vi "Initialize RF boards - interlace 3 v2.vi"(2 "error in":errorcluster, 3 "FPGA VI Reference In":T1) -> (0 "error out":errorcluster, 1 "FPGA VI Reference Out":T1)   [LabVIEW 2012]
uses:
  <vilib>/rvi/interface/nirviReadWriteControl/nirviReadWriteControl.xnode
  openfpgaref.8.6.ctl
  NiFpgaLv.dll
  <vilib>/Utility/error.llb/Error Cluster From Error Code.vi
  <vilib>/rvi/errors/niLvFpgaAdjustHostInterfaceError.vi
  FPGA Bitfiles/UHR-FleezersInst_FPGATarget_UHR-Fleezers_main_12.5_v1.lvbitx
  <vilib>/rvi/errors/niLvFpgaMergeErrorWithErrorCode.vi
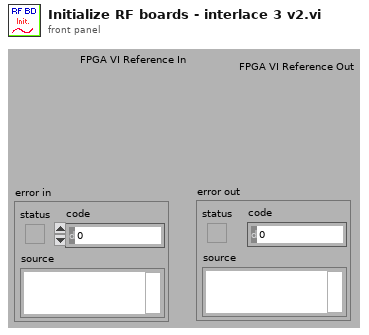
[diagram p1: front panel]
types:
  T1 = typedef "openfpgaref.8.6.ctl" = refnum<k20>
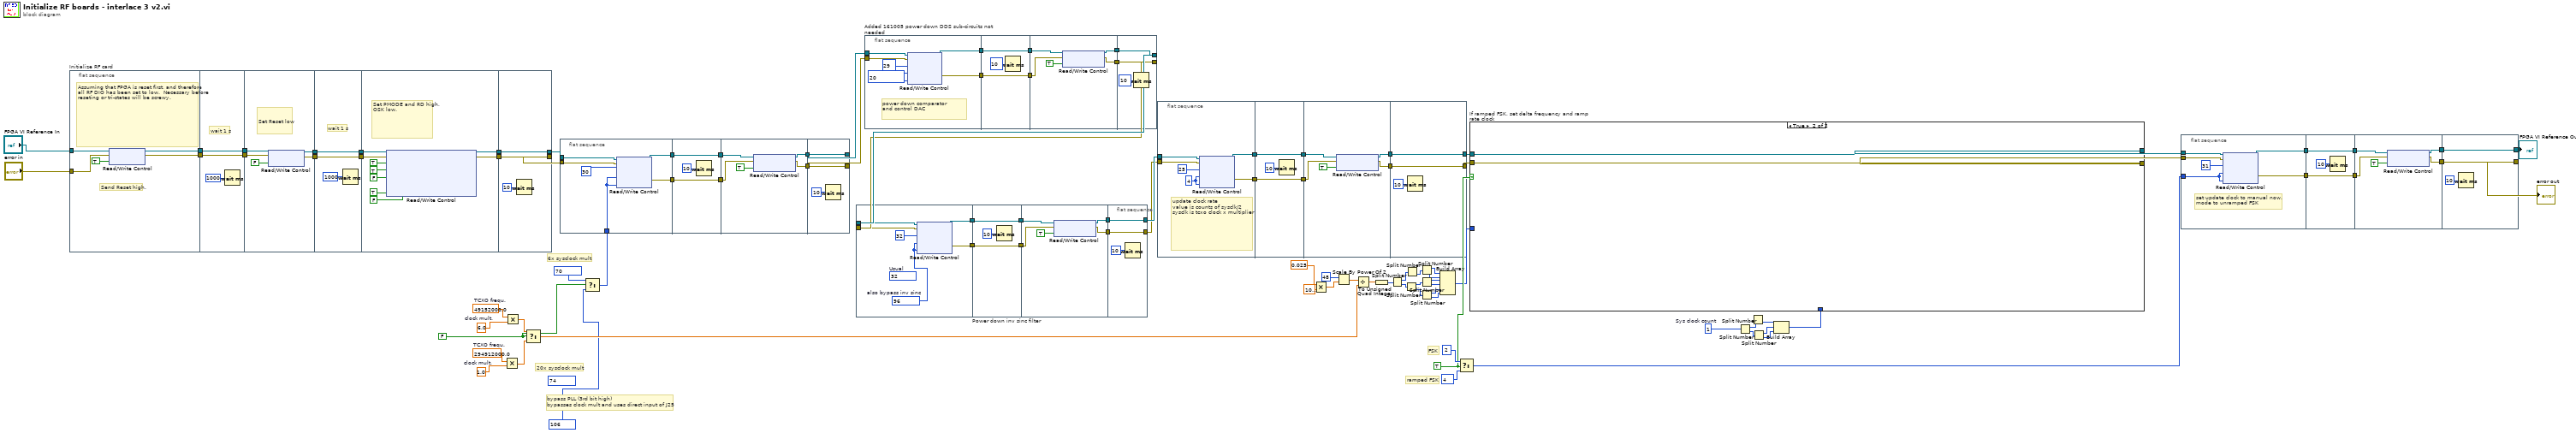
[diagram p0: block diagram]
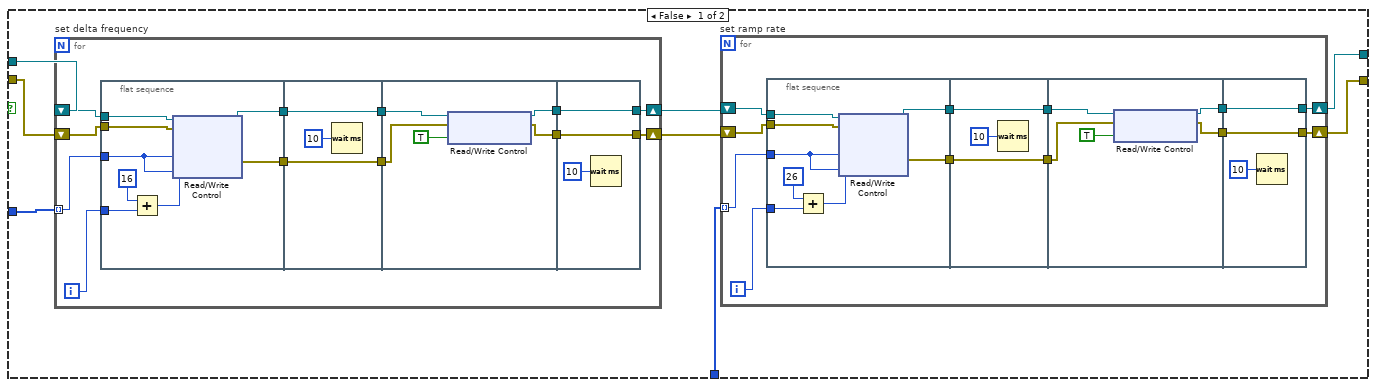
[diagram p2: hidden frame]
diagram:
  (unwired) u8 74 ("Data")
  w14 = FALSE ("s")
  w18 = 1.0  # clock mult.
  w17 = 294912000.0  # TCXO frequ.
  w21 = 6.0  # clock mult.
  w20 = 49152000.0  # TCXO frequ.
  w30 = u32 1  # Sys clock count
  w51 = TRUE
  # "bypass PLL (3rd bit high)\nbypasses clock mult and uses direct input of J25"
  # "20x sysclock mult"
  # "6x sysclock mult"
  # "ramped FSK"
  # "FSK"
  n1 = flat-sequence "Initialize RF card" {
    tunnel: [w102] -> w97
    tunnel: [w101] -> w96
    tunnel: "error in" -> [w100]
    tunnel: "FPGA VI Reference In" -> [w98]
    tunnel: w97 -> [w104]
    tunnel: w96 -> [w103]
    tunnel: [w104] -> w95
    tunnel: [w103] -> w94
    tunnel: w95 -> [w110]
    tunnel: w94 -> [w109]
    tunnel: [w108] -> w93
    tunnel: [w107] -> w92
    tunnel: w93 -> [w112]
    tunnel: w92 -> [w111]
    tunnel: [w112] -> w91
    tunnel: [w111] -> w90
    tunnel: w91 -> [w122]
    tunnel: w90 -> [w121]
    tunnel: [w118] -> w80
    tunnel: [w117] -> w79
    tunnel: [w124] -> w73
    tunnel: [w125] -> w74
    tunnel: w80 -> [w125]
    tunnel: w79 -> [w124]
    frame #0 {
      # "Send Reset high."
      # "Assuming that FPGA is reset first, and therefore\nall RF DIO has been set to low.  Necessary before\nreseting or tri-states will be screwy."
      n2 = xnode "Read/Write Control"("FPGA VI Reference In"=w98, "error in"=w100, "Reset Bd 1"=TRUE ("Reset")) -> ("FPGA VI Reference Out"=w102:T1, "error out"=w101:errorcluster)
    }
    frame #1 {
      # "wait 1 s"
      n3 = Wait (ms)(milliseconds to wait=u32 1000) -> ()  [unwired: 1 out]
    }
    frame #2 {
      # "Set Reset low"
      n4 = xnode "Read/Write Control"("FPGA VI Reference In"=w110, "error in"=w109, "Reset Bd 1"=FALSE ("Reset")) -> ("FPGA VI Reference Out"=w108:T1, "error out"=w107:errorcluster)
    }
    frame #3 {
      # "wait 1 s"
      n5 = Wait (ms)(milliseconds to wait=u32 1000) -> ()  [unwired: 1 out]
    }
    frame #4 {
      # "Set PMODE and RD high,\nOSK low."
      n6 = xnode "Read/Write Control"("FPGA VI Reference In"=w122, "error in"=w121, "RD"=TRUE, "PMODE"=TRUE, "OSK Bd 1"=FALSE ("OSK"), "Direct RF Box  Communication"=TRUE, "FPGA Controls  RF Box"=FALSE) -> ("FPGA VI Reference Out"=w118:T1, "error out"=w117:errorcluster)
    }
    frame #5 {
      n7 = Wait (ms)(milliseconds to wait=u32 10) -> ()  [unwired: 1 out]
    }
  }
  n8 = Multiply(x=w17, y=w18) -> (x*y=w16:dbl)
  n9 = Multiply(x=w20, y=w21) -> (x*y=w19:dbl)
  n10 = Select(t=w19, s=w14, f=w16) -> (s? t:f=w15:dbl)
  n11 = flat-sequence {
    tunnel: [w131] -> w89
    tunnel: [w130] -> w88
    tunnel: w74 -> [w129]
    tunnel: w73 -> [w128]
    tunnel: w12 -> [w126]
    tunnel: [w133] -> w87
    tunnel: w89 -> [w133]
    tunnel: [w132] -> w86
    tunnel: w88 -> [w132]
    tunnel: w87 -> [w139]
    tunnel: w86 -> [w138]
    tunnel: [w136] -> w78
    tunnel: [w135] -> w77
    tunnel: [w141] -> w3
    tunnel: [w142] -> w4
    tunnel: w78 -> [w142]
    tunnel: w77 -> [w141]
    frame #0 {
      n12 = xnode "Read/Write Control"("FPGA VI Reference In"=w129, "error in"=w128, "Address"=u8 30, "Data BD 1"=w126, "Data BD 2"=w126) -> ("FPGA VI Reference Out"=w131:T1, "error out"=w130:errorcluster)
    }
    frame #1 {
      n13 = Wait (ms)(milliseconds to wait=u32 10) -> ()  [unwired: 1 out]
    }
    frame #2 {
      n14 = xnode "Read/Write Control"("FPGA VI Reference In"=w139, "error in"=w138, "Update Data"=TRUE) -> ("FPGA VI Reference Out"=w136:T1, "error out"=w135:errorcluster)
    }
    frame #3 {
      n15 = Wait (ms)(milliseconds to wait=u32 10) -> ()  [unwired: 1 out]
    }
  }
  n16 = Select(t=u8 70 ("Data"), s=w14, f=u8 106 ("Data")) -> (s? t:f=w12:u8)
  n17 = flat-sequence "Power down inv sinc filter" {
    tunnel: [w148] -> w85
    tunnel: [w147] -> w84
    tunnel: w2 -> [w146]
    tunnel: w1 -> [w145]
    tunnel: [w150] -> w83
    tunnel: w85 -> [w150]
    tunnel: [w149] -> w82
    tunnel: w84 -> [w149]
    tunnel: w83 -> [w156]
    tunnel: w82 -> [w155]
    tunnel: [w153] -> w76
    tunnel: [w152] -> w75
    tunnel: [w158] -> w65
    tunnel: [w159] -> w66
    tunnel: w76 -> [w159]
    tunnel: w75 -> [w158]
    frame #0 {
      w143 = u8 96  # also bypass inv sinc
      (unwired) u8 32  # Usual
      n18 = xnode "Read/Write Control"("FPGA VI Reference In"=w146, "error in"=w145, "Address"=u8 32, "Data BD 1"=w143, "Data BD 2"=w143) -> ("FPGA VI Reference Out"=w148:T1, "error out"=w147:errorcluster)
    }
    frame #1 {
      n19 = Wait (ms)(milliseconds to wait=u32 10) -> ()  [unwired: 1 out]
    }
    frame #2 {
      n20 = xnode "Read/Write Control"("FPGA VI Reference In"=w156, "error in"=w155, "Update Data"=TRUE) -> ("FPGA VI Reference Out"=w153:T1, "error out"=w152:errorcluster)
    }
    frame #3 {
      n21 = Wait (ms)(milliseconds to wait=u32 10) -> ()  [unwired: 1 out]
    }
  }
  n22 = flat-sequence "Added 161005 power down DDS sub-circuits not needed" {
    tunnel: [w165] -> w10
    tunnel: [w164] -> w9
    tunnel: w4 -> [w163]
    tunnel: w3 -> [w162]
    tunnel: [w167] -> w8
    tunnel: w10 -> [w167]
    tunnel: [w166] -> w7
    tunnel: w9 -> [w166]
    tunnel: w8 -> [w173]
    tunnel: w7 -> [w172]
    tunnel: [w170] -> w6
    tunnel: [w169] -> w5
    tunnel: [w176] -> w1
    tunnel: w6 -> [w174]
    tunnel: w5 -> [w176]
    tunnel: [w174] -> w2
    frame #0 {
      w160 = u8 20 ("Data")
      # "power down comparator\nand control DAC"
      n23 = xnode "Read/Write Control"("FPGA VI Reference In"=w163, "error in"=w162, "Address"=u8 29, "Data BD 1"=w160, "Data BD 2"=w160) -> ("FPGA VI Reference Out"=w165:T1, "error out"=w164:errorcluster)
    }
    frame #1 {
      n24 = Wait (ms)(milliseconds to wait=u32 10) -> ()  [unwired: 1 out]
    }
    frame #2 {
      n25 = xnode "Read/Write Control"("FPGA VI Reference In"=w173, "error in"=w172, "Update Data"=TRUE) -> ("FPGA VI Reference Out"=w170:T1, "error out"=w169:errorcluster)
    }
    frame #3 {
      n26 = Wait (ms)(milliseconds to wait=u32 10) -> ()  [unwired: 1 out]
    }
  }
  n27 = flat-sequence {
    tunnel: [w182] -> w72
    tunnel: [w181] -> w71
    tunnel: w66 -> [w180]
    tunnel: w65 -> [w179]
    tunnel: [w184] -> w70
    tunnel: w72 -> [w184]
    tunnel: [w183] -> w69
    tunnel: w71 -> [w183]
    tunnel: w70 -> [w190]
    tunnel: w69 -> [w189]
    tunnel: [w187] -> w68
    tunnel: [w186] -> w67
    tunnel: [w192] -> w63
    tunnel: [w193] -> w64
    tunnel: w68 -> [w193]
    tunnel: w67 -> [w192]
    frame #0 {
      w177 = u8 4 ("Data")
      # "update clock rate\nvalue is counts of sysclk/2\nsysclk is tcxo clock x multiplier"
      n28 = xnode "Read/Write Control"("FPGA VI Reference In"=w180, "error in"=w179, "Address"=u8 25, "Data BD 1"=w177, "Data BD 2"=w177) -> ("FPGA VI Reference Out"=w182:T1, "error out"=w181:errorcluster)
    }
    frame #1 {
      n29 = Wait (ms)(milliseconds to wait=u32 10) -> ()  [unwired: 1 out]
    }
    frame #2 {
      n30 = xnode "Read/Write Control"("FPGA VI Reference In"=w190, "error in"=w189, "Update Data"=TRUE) -> ("FPGA VI Reference Out"=w187:T1, "error out"=w186:errorcluster)
    }
    frame #3 {
      n31 = Wait (ms)(milliseconds to wait=u32 10) -> ()  [unwired: 1 out]
    }
  }
  n32 = Multiply(x=0.025 ("Delta Frequency  (MHz)"), y=1000000.0) -> (x*y=w46:dbl)
  n33 = Scale By Power Of 2(n=48, x=w46) -> (x*2^n=w48:dbl)
  n34 = Divide(x=w48, y=w15) -> (x/y=w47:dbl)
  n35 = To Unsigned Quad Integer(1:w47) -> (0:w43:u64)
  n36 = Split Number(x=w43) -> (hi(x)=w42:u32, lo(x)=w41:u32)
  n37 = Split Number(x=w41) -> (hi(x)=w39:u16, lo(x)=w40:u16)
  n38 = Split Number(x=w42) -> (lo(x)=w38:u16)  [unwired: 1 out]
  n39 = Split Number(x=w38) -> (hi(x)=w37:u8, lo(x)=w36:u8)
  n40 = Split Number(x=w39) -> (hi(x)=w35:u8, lo(x)=w34:u8)
  n41 = Split Number(x=w40) -> (hi(x)=w33:u8, lo(x)=w32:u8)
  n42 = Build Array(w37, w36, w35, w34, w33, w32) -> (w31:u8[])
  n43 = Select(t=u8 2 ("Data"), s=w51, f=u8 4 ("Data")) -> (s? t:f=w52:u8)
  n44 = Split Number(x=w30) -> (hi(x)=w29:u16, lo(x)=w28:u16)
  n45 = Split Number(x=w29) -> (lo(x)=w27:u8)  [unwired: 1 out]
  n46 = Split Number(x=w28) -> (hi(x)=w26:u8, lo(x)=w25:u8)
  n47 = Build Array(w27, w26, w25) -> (w24:u8[])
  n48 = case "If ramped FSK, set delta frequency and ramp rate clock" shown="True" w51 {
    tunnel: w64 -> [w201 w265]
    tunnel: w63 -> [w200 w264]
    tunnel: [w195 w264] -> w60
    tunnel: [w196 w265] -> w59
    tunnel: w31 -> [w199 _]
    tunnel: w24 -> [w194 _]
    frame False {
      n49 = for "set delta frequency" {
        shift-right: [w235] -> w198
        shift-left: w201 -> [w238]
        shift-right: [w236] -> w197
        shift-left: w200 -> [w237]
        tunnel: w199 -> [w233] mode=indexing
        i -> [w234]
        n50 = flat-sequence {
          tunnel: [w252] -> w244
          tunnel: [w251] -> w243
          tunnel: w238 -> [w250]
          tunnel: w237 -> [w249]
          tunnel: w234 -> [w247]
          tunnel: w233 -> [w245]
          tunnel: [w254] -> w242
          tunnel: w244 -> [w254]
          tunnel: [w253] -> w241
          tunnel: w243 -> [w253]
          tunnel: w242 -> [w260]
          tunnel: w241 -> [w259]
          tunnel: [w257] -> w240
          tunnel: [w256] -> w239
          tunnel: [w263] -> w236
          tunnel: [w261] -> w235
          tunnel: w240 -> [w261]
          tunnel: w239 -> [w263]
          frame #0 {
            n51 = Add(x=u8 16 ("Address"), y=w247) -> (x+y=w246:i32)
            n52 = xnode "Read/Write Control"("FPGA VI Reference In"=w250, "error in"=w249, "Address"=w246, "Data BD 1"=w245, "Data BD 2"=w245) -> ("FPGA VI Reference Out"=w252:T1, "error out"=w251:errorcluster)
          }
          frame #1 {
            n53 = Wait (ms)(milliseconds to wait=u32 10) -> ()  [unwired: 1 out]
          }
          frame #2 {
            n54 = xnode "Read/Write Control"("FPGA VI Reference In"=w260, "error in"=w259, "Update Data"=TRUE) -> ("FPGA VI Reference Out"=w257:T1, "error out"=w256:errorcluster)
          }
          frame #3 {
            n55 = Wait (ms)(milliseconds to wait=u32 10) -> ()  [unwired: 1 out]
          }
        }
      }
      n56 = for "set ramp rate" {
        shift-right: [w204] -> w196
        shift-left: w198 -> [w207]
        shift-right: [w205] -> w195
        shift-left: w197 -> [w206]
        tunnel: w194 -> [w202] mode=indexing
        i -> [w203]
        n57 = flat-sequence {
          tunnel: [w221] -> w213
          tunnel: [w220] -> w212
          tunnel: w207 -> [w219]
          tunnel: w206 -> [w218]
          tunnel: w203 -> [w216]
          tunnel: w202 -> [w214]
          tunnel: [w223] -> w211
          tunnel: w213 -> [w223]
          tunnel: [w222] -> w210
          tunnel: w212 -> [w222]
          tunnel: w211 -> [w229]
          tunnel: w210 -> [w228]
          tunnel: [w226] -> w209
          tunnel: [w225] -> w208
          tunnel: [w232] -> w205
          tunnel: [w230] -> w204
          tunnel: w209 -> [w230]
          tunnel: w208 -> [w232]
          frame #0 {
            n58 = Add(x=u8 26 ("Address"), y=w216) -> (x+y=w215:i32)
            n59 = xnode "Read/Write Control"("FPGA VI Reference In"=w219, "error in"=w218, "Address"=w215, "Data BD 1"=w214, "Data BD 2"=w214) -> ("FPGA VI Reference Out"=w221:T1, "error out"=w220:errorcluster)
          }
          frame #1 {
            n60 = Wait (ms)(milliseconds to wait=u32 10) -> ()  [unwired: 1 out]
          }
          frame #2 {
            n61 = xnode "Read/Write Control"("FPGA VI Reference In"=w229, "error in"=w228, "Update Data"=TRUE) -> ("FPGA VI Reference Out"=w226:T1, "error out"=w225:errorcluster)
          }
          frame #3 {
            n62 = Wait (ms)(milliseconds to wait=u32 10) -> ()  [unwired: 1 out]
          }
        }
      }
    }
    frame True {
    }
  }
  n63 = flat-sequence {
    tunnel: [w271] -> w58
    tunnel: [w270] -> w57
    tunnel: w59 -> [w269]
    tunnel: w60 -> [w268]
    tunnel: w52 -> [w266]
    tunnel: [w273] -> w56
    tunnel: w58 -> [w273]
    tunnel: [w272] -> w55
    tunnel: w57 -> [w272]
    tunnel: w56 -> [w279]
    tunnel: w55 -> [w278]
    tunnel: [w276] -> w54
    tunnel: [w275] -> w53
    tunnel: [w281] -> w50
    tunnel: [w282] -> w23
    tunnel: w54 -> [w282]
    tunnel: w53 -> [w281]
    frame #0 {
      # "set update clock to manual now,\nmode to unramped FSK"
      n64 = xnode "Read/Write Control"("FPGA VI Reference In"=w269, "error in"=w268, "Address"=u8 31, "Data BD 1"=w266, "Data BD 2"=w266) -> ("FPGA VI Reference Out"=w271:T1, "error out"=w270:errorcluster)
    }
    frame #1 {
      n65 = Wait (ms)(milliseconds to wait=u32 10) -> ()  [unwired: 1 out]
    }
    frame #2 {
      n66 = xnode "Read/Write Control"("FPGA VI Reference In"=w279, "error in"=w278, "Update Data"=TRUE) -> ("FPGA VI Reference Out"=w276:T1, "error out"=w275:errorcluster)
    }
    frame #3 {
      n67 = Wait (ms)(milliseconds to wait=u32 10) -> ()  [unwired: 1 out]
    }
  }
  "error out" <- w50
  "FPGA VI Reference Out" <- w23
